vi "PPG_ABC.wait until not running.vi"(0 "i ref in":refnum<vi>, 3 "ms timeout (10000)":i32=10000, 5 "error in (no error)":errorcluster) -> (14 "i ref out":refnum<vi>, 17 "timed out":bool, 19 "error out":errorcluster)   [LabVIEW 2014, in "PPG_ABC.lvlib"]
doc: "Waits until pattern execution is no longer in progress. This method called only from the \"load ABC\" method to delay the loading of patterns until pattern execution has finished."
uses:
  PPG_ABC.lvlib
  PPG_ABC.PG_Running.ctl
  CSCore/CSSystem/CoreDefs/CoreDefs.error_type.ctl
  CSCore/CSSystem/CoreDefs/CoreDefs.error_severity.ctl
  CSCore/CSSystem/CoreLib/CoreLib.lvlib
  CSlibraries/UtilityLib/UtilityLib.lvlib
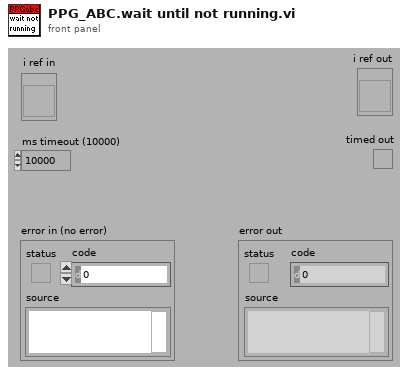
[diagram p1: front panel]
types:
  T1 = typedef "CoreDefs.error_severity.ctl" = enum16{"undefined", "information", "warning", "error", "fatal"}
  T2 = typedef "CoreDefs.error_type.ctl" = enum16{"no error", "can't load process", "can't unload process", "process does not exist", "can't install process", "can't remove process", "unknown function", "time out", "can't execute function", "duplicate queue name", "super not found", "caller queue invalid", "can't ping process", "unknown error", "VISA Error", "VISA timeout", "GPIB timeout", "GPIB error", "communication error", "data type mismatch", "can't read data from OPC server", "can't write data to OPC server", "OET error", "function not implemented", "process already exists", "invalid Shared Variable name", "error writing Shared Variable", "error reading Shared Variable", "invalid client name", "corrupt database", "unknown class", "call not authorized", "parameter out of range", "OET timeout: can't get data to modify", "invalid queue name", "requested operation incompatible with current state", "event undefined", "event disabled", "state undefined", "caller is not a friend", "EventBuilder: bad eventID", "EventBuilder: no DAQ devices", "a thread must not stop itself", "UNUSED ELEMENT4", "DiscArchiver: eventData incomplete", "DiscArchiver: eventData does not belong to run", "DiscArchiver: can't open file", "DiscArchiver: can't write to file", "DiscArchiver: available disc space low", "can't acquire semaphore", "error reading data from database", "notifier object is not existing", "can't register process", "can't unregister process", "illegal event type", "object disabled", "object already exists", "can't change state", "Instrument not found", "no connection to remote node", "invalid reference", "N/A", "UNUSED ELEMENT 1", "element not found", "illegal TCP/IP connection detected", "object does not exist", "invalid access ID", "unknown CS system", "invalid privilige", "unsupported data type", "unsupported server type", "IO server already exists", "Shared Variable already exists"}
  T3 = typedef "PPG_ABC.lvlib/PPG_ABC.PG_Running.ctl" = i32
  T4 = typedef "PPG_ABC.lvlib/PPG_ABC.i attribute.ctl" = cluster{"patternGroups":T5[], "defaultLetter":string, "defaultPatternGroup":i32, "PGRunning":T3, "PGRunningID":i32, "pgStarting":T6}
  T5 = typedef "PPG_ABC.lvlib/PPG_ABC.PG_dataType.ctl" = cluster{"PGDevice":string, "rawPatternData":cluster{"triggerCondition":i32, "timeTable":dbl[], "channelTable":string[]}[]}
  T6 = typedef "Semaphore RefNum" = refnum<k1>
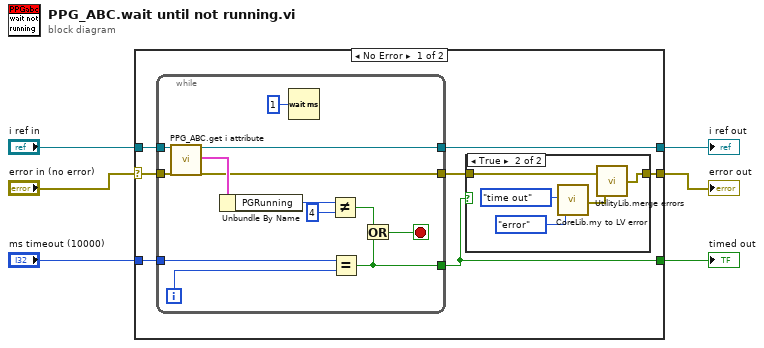
[diagram p0: block diagram]
diagram:
  n1 = case shown="No Error" "error in (no error)" {
    selector: "error in (no error)" -> [w12 w33]
    tunnel: "i ref in" -> [w13 w34]
    tunnel: [w10 w34] -> w4
    tunnel: [w7 w33] -> w3
    tunnel: "ms timeout (10000)" -> [w11 _]
    tunnel: [w9 _] -> w1
    frame No Error {
      n2 = while {
        tunnel: w13 -> [w31]
        tunnel: w12 -> [w30]
        tunnel: w11 -> [w25]
        tunnel: [w22] -> w9
        tunnel: [w21] -> w10
        tunnel: [w20] -> w8
        i -> [w26]
        stop <- w23 stop-if-true
        n3 = call "PPG_ABC.get i attribute.vi"("i ref in"=w31, "error in (no error)"=w30) -> ("i ref out"=w21:refnum<vi>, "i attribute"=w32:T4, "error out"=w20:errorcluster)  [unwired: 15 in]
        n4 = Unbundle By Name(w32) -> ("PGRunning"=w29:T3)
        n5 = Wait (ms)(milliseconds to wait=u32 1) -> ()  [unwired: 1 out]
        n6 = Not Equal?(x=w29, y=T3 4) -> (x != y?=w24:bool)
        n7 = Equal?(x=w25, y=w26) -> (x = y?=w22:bool)
        n8 = Or(x=w24, y=w22) -> (x .or. y?=w23:bool)
      }
      n9 = case shown="True" w9 {
        tunnel: w8 -> [w14 w17]
        tunnel: [w14 w15] -> w7
        frame False {
        }
        frame True {
          n10 = call "CoreLib.my to LV error.vi"("ErrorTypes"=CoreDefs.error_type."time out", "severityLevel"=CoreDefs.error_severity."error") -> ("myErrorCluster"=w16:errorcluster)  [unwired: 16 in, 1 out]
          n11 = call "UtilityLib.merge errors.vi"("error2 (no error)"=w16, "error1 (no error)"=w17) -> ("error out"=w15:errorcluster)
        }
      }
    }
    frame Error {
    }
  }
  "error out" <- w3
  "i ref out" <- w4
  "timed out" <- w1
